vi "Memory.Pointer.Bool.New.vi"(8 "error in (no error)":errorcluster) -> (0 "error out":errorcluster, 3 "Bool Pointer":refnum<class "Memory.Pointer.Bool.lvclass">)   [LabVIEW 2016, in "Memory Manager.lvlib" / "Memory.Pointer.Bool.lvclass"]
doc: "Allocates a new block of memory, represented by Pointer."
uses:
  Memory.Pointer.Bool.lvclass
  C:/Users/Ryan/Documents/Git/Sourcetree/LabVIEW-Memory-Manager/Source/Library/Classes/Pointer/Pointer.Void/Memory.Pointer.Void.lvclass
  Pointer.Void/Memory.Pointer.Void.lvclass/Memory.Pointer.Void.ctl
  Pointer.Void/Methods/Memory.Pointer.Set Address.vi
  Pointer.Void/Methods/Memory.Pointer.Get Size.vi
  Pointer.Void/Memory.Pointer.Void.lvclass
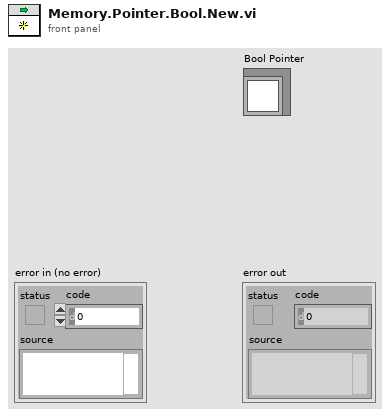
[diagram p1: front panel]
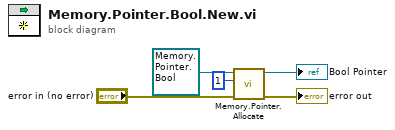
[diagram p0: block diagram]
diagram:
  n1 = call "Memory.Pointer.Allocate.vi"("error in (no error)"="error in (no error)", "allocation limit (0x7FFFFFFF: 2GiB)"=u64 1 ("size"), "Pointer in"=refnum<class "Memory.Pointer.Bool.lvclass"> refnum ("LabVIEW Memory Manager.lvlib:DBL Pointer")) -> ("error out"=→"error out":errorcluster, "Pointer out"=→"Bool Pointer":refnum<class "Memory.Pointer.Bool.lvclass">)  [unwired: 6 in, 1 out]
